vi "TalonMotionMagic.vi"(1 "error out":errorcluster, 2 "Numeric Value Inputs":T1, 3 "Boolean Value Inputs":T2, 4 "xMotorControlDevRef":T3={"DeviceStatus"={"status"=FALSE, "code"=0, "source"=""}, "Type"=enum."PWM", "PWM"={"PWM Channel"=enum."Invalid", "DeadBand"={"Name"="", "maxPositivePwm"=0, "minPositivePwm"=0, "centerPwm"=0, "maxNegativePwm"=0, "minNegativePwm"=0, "angularRange"=0}}, "CAN"={"Device Number"=0, "SetOutput VI Ref"=variant, "GetOutput VI Ref"=variant, "Enable VI Ref"=variant, "Disable VI Ref"=variant, "Data"=variant}, "Invert"=FALSE, "DIO PWM"={"PWM \"Enable\" Channel"=enum."Invalid", "DIOChannel"=enum."Invalid", "PWM Rate"=0.0}}) -> (0 "Graph Output":cluster{"Hood Setpoint":dbl, dbl})   [LabVIEW 2020]
uses:
  TitanLib/Lib/TitanLib.lvlib
  <vilib>/Rock Robotics/WPI/ThirdParty/Phoenix-LabVIEW/Motor Controller/Controls/CTRE_Phoenix_MotorControl_ControlMode.ctl
  <vilib>/Rock Robotics/WPI/ThirdParty/Phoenix-LabVIEW/Motor Controller/Get/CTRE_Phoenix_MotorController_GetSelectedSensorData.vi
  <vilib>/Rock Robotics/SystemInterfaces/DIO/FPGA_DIOPWMChannel.ctl
  <vilib>/Rock Robotics/WPI/PWM/WPI_PWMDeadband.ctl
  <vilib>/Rock Robotics/WPI/MotorControl/WPI_MotorControlType.ctl
  <vilib>/Rock Robotics/SystemInterfaces/DIO/FPGA_DIOChannel.ctl
  <vilib>/Rock Robotics/WPI/MotorControl/WPI_MotorControlDeviceRef.ctl
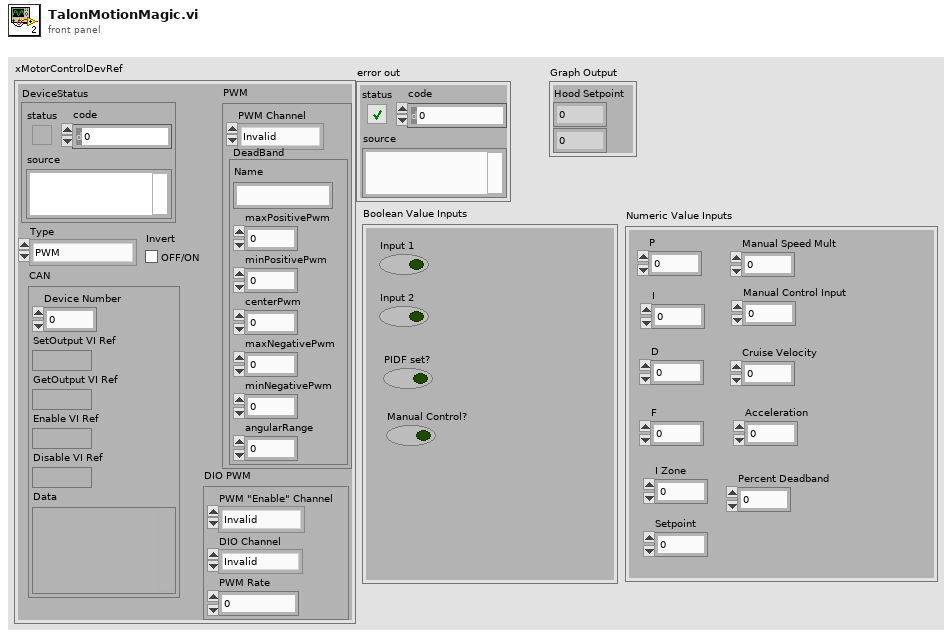
[diagram p1: front panel]
types:
  T1 = cluster{"P":dbl, "I":dbl, "D":dbl, "F":dbl, "I Zone":dbl, "Setpoint":dbl, "Manual Speed Mult":dbl, "Manual Control Input":dbl, "Cruise Velocity":i32, "Acceleration":i32, "Percent Deadband":dbl}
  T2 = cluster{"Input 1":bool, "Input 2":bool, "PIDF set?":bool, "Manual Control?":bool}
  T3 = typedef "WPI_MotorControlDeviceRef.ctl" = cluster{"DeviceStatus":errorcluster, "Type":T4, "PWM":cluster{"PWM Channel":T5, "DeadBand":T6}, "CAN":cluster{"Device Number":u8, "SetOutput VI Ref":variant, "GetOutput VI Ref":variant, "Enable VI Ref":variant, "Disable VI Ref":variant, "Data":variant}, "Invert":bool, "DIO PWM":cluster{"PWM \"Enable\" Channel":T5, "DIOChannel":T7, "PWM Rate":dbl}}
  T4 = typedef "WPI_MotorControlType.ctl" = enum16{"PWM", "CAN", "DIO PWM"}
  T5 = typedef "FPGA_DIOPWMChannel.ctl" = enum8{"PWM 0", "PWM 1", "PWM 2", "PWM 3", "PWM 4", "PWM 5", "PWM 6", "PWM 7", "PWM 8", "PWM 9", "PWM MXP 0", "PWM MXP 1", "PWM MXP 2", "PWM MXP 3", "PWM MXP 4", "PWM MXP 5", "PWM MXP 6", "PWM MXP 7", "PWM MXP 8", "PWM MXP 9", "Invalid"}
  T6 = typedef "WPI_PWMDeadband.ctl" = cluster{"Name":string, "maxPositivePwm":i32, "minPositivePwm":i32, "centerPwm":i32, "maxNegativePwm":i32, "minNegativePwm":i32, "angularRange":u16}
  T7 = typedef "FPGA_DIOChannel.ctl" = enum8{"DIO 0", "DIO 1", "DIO 2", "DIO 3", "DIO 4", "DIO 5", "DIO 6", "DIO 7", "DIO 8", "DIO 9", "DIO MXP 0", "DIO MXP 1", "DIO MXP 2", "DIO MXP 3", "DIO MXP 4", "DIO MXP 5", "DIO MXP 6", "DIO MXP 7", "DIO MXP 8", "DIO MXP 9", "DIO MXP 10", "DIO MXP 11", "DIO MXP 12", "DIO MXP 13", "DIO MXP 14", "DIO MXP 15", "SPI Port CS1", "SPI Port CS2", "SPI Port CS3", "SPI Port MISO", "SPI Port MOSI", "Invalid"}
  T8 = typedef "CTRE_Phoenix_MotorControl_ControlMode.ctl" = u16
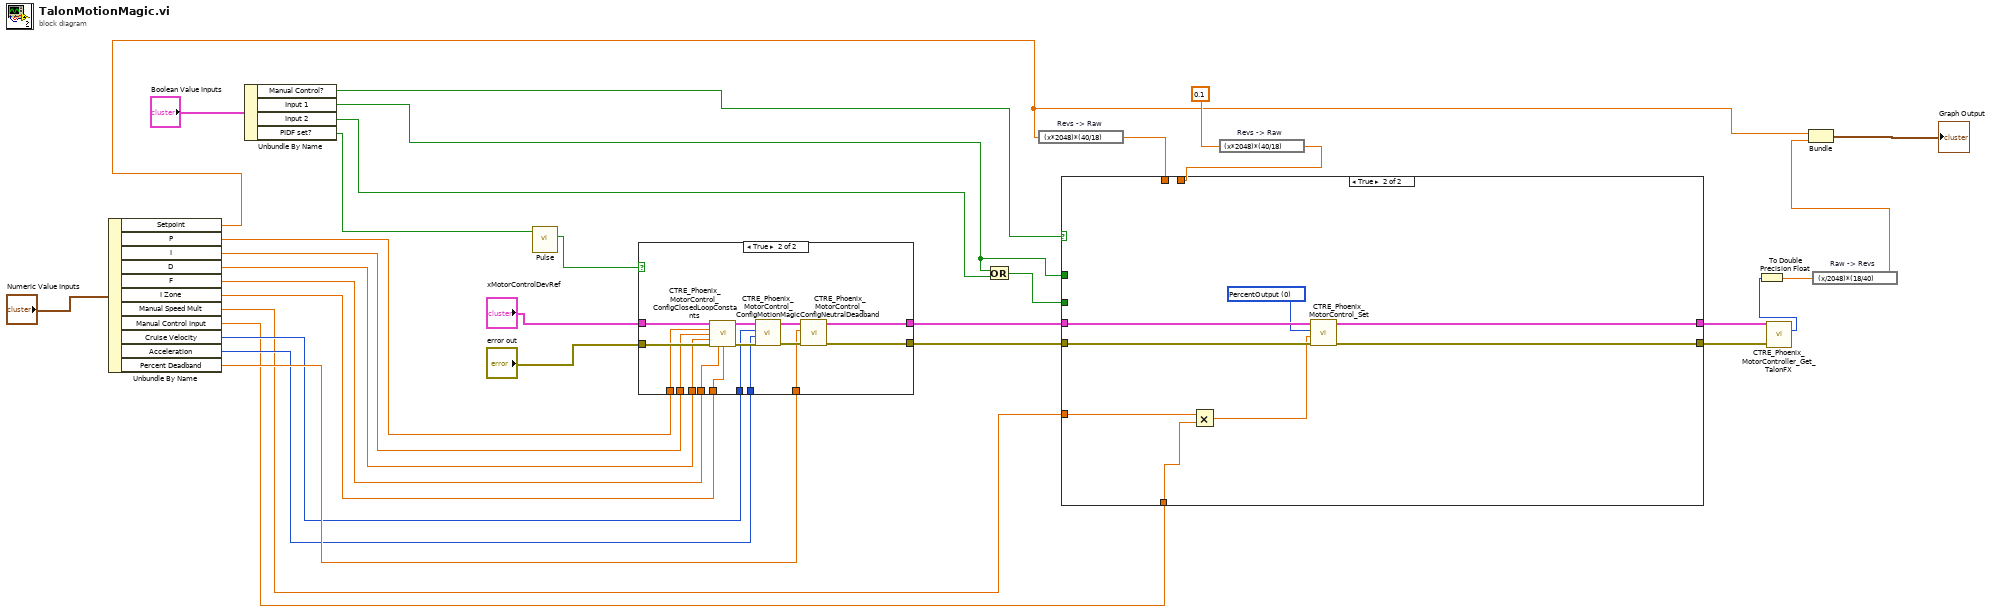
[diagram p0: block diagram]
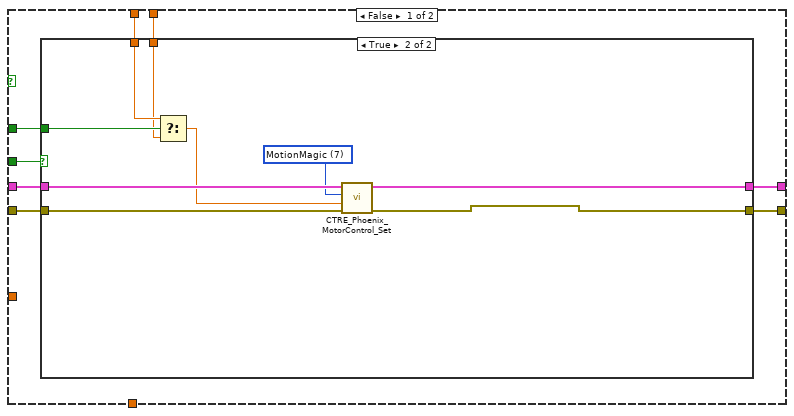
[diagram p2: hidden frame]
diagram:
  n1 = Unbundle By Name("Numeric Value Inputs") -> ("Setpoint"=w11:dbl, "P"=w10:dbl, "I"=w9:dbl, "D"=w8:dbl, "F"=w7:dbl, "I Zone"=w6:dbl, "Manual Speed Mult"=w2:dbl, "Manual Control Input"=w1:dbl, "Cruise Velocity"=w4:i32, "Acceleration"=w3:i32, "Percent Deadband"=w5:dbl)
  n2 = Unbundle By Name("Boolean Value Inputs") -> ("Manual Control?"=w13:bool, "Input 1"=w14:bool, "Input 2"=w15:bool, "PIDF set?"=w16:bool)
  n3 = call "Pulse.vi"("Input"=w16) -> ("Output"=w20:bool)  [unwired: 10 in]
  n4 = case shown="True" w20 {
    tunnel: "xMotorControlDevRef" -> [w34 w50]
    tunnel: "error out" -> [w33 w49]
    tunnel: w10 -> [_ w48]
    tunnel: w9 -> [_ w47]
    tunnel: w8 -> [_ w46]
    tunnel: w7 -> [_ w45]
    tunnel: w6 -> [_ w44]
    tunnel: w4 -> [_ w41]
    tunnel: w3 -> [_ w40]
    tunnel: w5 -> [_ w37]
    tunnel: [w34 w36] -> w21
    tunnel: [w33 w35] -> w22
    frame False {
    }
    frame True {
      n5 = call <vilib>:"CTRE_Phoenix_MotorControl_ConfigClosedLoopConstants.vi"("PhoenixMotorControlDevRef"=w50, "P"=w48, "I"=w47, "D"=w46, "error in (no error)"=w49, "F"=w45, "I Zone"=w44) -> ("PhoenixMotorControlDevRef"=w42:T3, "error out"=w43:errorcluster)  [unwired: 7 in]
      n6 = call <vilib>:"CTRE_Phoenix_MotorControl_ConfigMotionMagic.vi"("error in (no error)"=w43, "Acceleration"=w40, "Cruise Velocity"=w41, "PhoenixMotorControlDevRef"=w42) -> ("error out"=w39:errorcluster, "PhoenixMotorControlDevRef"=w38:T3)  [unwired: 6 in]
      n7 = call <vilib>:"CTRE_Phoenix_MotorControl_ConfigNeutralDeadband.vi"("error in (no error)"=w39, "Percent Deadband"=w37, "PhoenixMotorControlDevRef"=w38) -> ("error out"=w35:errorcluster, "PhoenixMotorControlDevRef"=w36:T3)  [unwired: 7 in]
    }
  }
  n8 = Or(x=w14, y=w15) -> (x .or. y?=w23:bool)
  n9 = expression code="(x*2048)*(40/18)" "Revs -> Raw"(w11) -> (w30:dbl)
  n10 = expression code="(x*2048)*(40/18)" "Revs -> Raw"(0.1 ("Max (deg)")) -> (w28:dbl)
  n11 = case shown="True" w13 {
    tunnel: w21 -> [w58 w77]
    tunnel: w22 -> [w57 w76]
    tunnel: w23 -> [w56 _]
    tunnel: w14 -> [w55 _]
    tunnel: w30 -> [w54 _]
    tunnel: w28 -> [w53 _]
    tunnel: w2 -> [_ w75]
    tunnel: [w52 w72] -> w24
    tunnel: [w51 w71] -> w25
    tunnel: w1 -> [_ w70]
    frame False {
      n12 = case shown="True" w56 {
        tunnel: w58 -> [w60 w69]
        tunnel: w57 -> [w59 w68]
        tunnel: w55 -> [_ w66]
        tunnel: w54 -> [_ w64]
        tunnel: w53 -> [_ w63]
        tunnel: [w60 w62] -> w52
        tunnel: [w59 w61] -> w51
        frame False {
        }
        frame True {
          w67 = T8 7 items=["PercentOutput"=0, "Position"=1, "Velocity"=2, "Current"=3, "Follower"=5, "MotionProfile"=6, "MotionMagic"=7, "MotionProfileArc"=10, "Disabled"=15] ("Control Mode")
          n13 = Select(t=w64, s=w66, f=w63) -> (s? t:f=w65:dbl)
          n14 = call <vilib>:"CTRE_Phoenix_MotorControl_Set.vi"("error in (no error)"=w68, "Output"=w65, "Control Mode"=w67, "PhoenixMotorControlDevRef"=w69) -> ("error out"=w61:errorcluster, "PhoenixMotorControlDevRef"=w62:T3)  [unwired: 6 in]
        }
      }
    }
    frame True {
      w73 = T8 0 items=["PercentOutput"=0, "Position"=1, "Velocity"=2, "Current"=3, "Follower"=5, "MotionProfile"=6, "MotionMagic"=7, "MotionProfileArc"=10, "Disabled"=15] ("Control Mode")
      n15 = Multiply(x=w75, y=w70) -> (x*y=w74:dbl)
      n16 = call <vilib>:"CTRE_Phoenix_MotorControl_Set.vi"("error in (no error)"=w76, "Output"=w74, "Control Mode"=w73, "PhoenixMotorControlDevRef"=w77) -> ("error out"=w71:errorcluster, "PhoenixMotorControlDevRef"=w72:T3)  [unwired: 6 in]
    }
  }
  n17 = call-poly <vilib>:"CTRE_Phoenix_MotorController_Get_TalonFX.vi"("PhoenixMotorControlDevRef"=w24, "error in"=w25) -> ("Position (Raw Sensor Units)"=w26:i32)  [unwired: 10 in, 3 out]
  n18 = To Double Precision Float(number=w26) -> (double precision float=w27:dbl)
  n19 = expression code="(x/2048)*(18/40)" "Raw -> Revs"(w27) -> (w31:dbl)
  n20 = Bundle("Setpoint"=w11, w31) -> (→"Graph Output":cluster{"Setpoint":dbl, dbl})  [unwired: 1 in]
